vi "更新程序.vi"() -> ()   [LabVIEW 2016, in "数据传输系统-02.lvlib" / "自动更新.lvlib"]
uses:
  <vilib>/FTP/NI_FTP.lvlib
panel:
  out "同名app个数":i32
  out "对比MD5":string
  out "当前MD5":string
  out "FTP链接结束":bool
  out "updateconfiguration":T1
  out "软件版本 2":string caption="目标软件版本"
  out "软件版本":string caption="当前软件版本"
  out "下载的文件名":string
  out "目标文件夹名":string
  out "端口号":i32
  out "IP地址":string
  out "步骤":string
  out "枚举":T2(ring)
  in  "目标路径（使用对话框）":path
  out "下载保存目录":path
  out "更新进度":u8(slide) scale=0.0..100.0
  # "1.下载更新--------2.MD5校验-------2.关闭主应用-------3.替换应用--------4.打开主应用-----------5.关闭本程序"
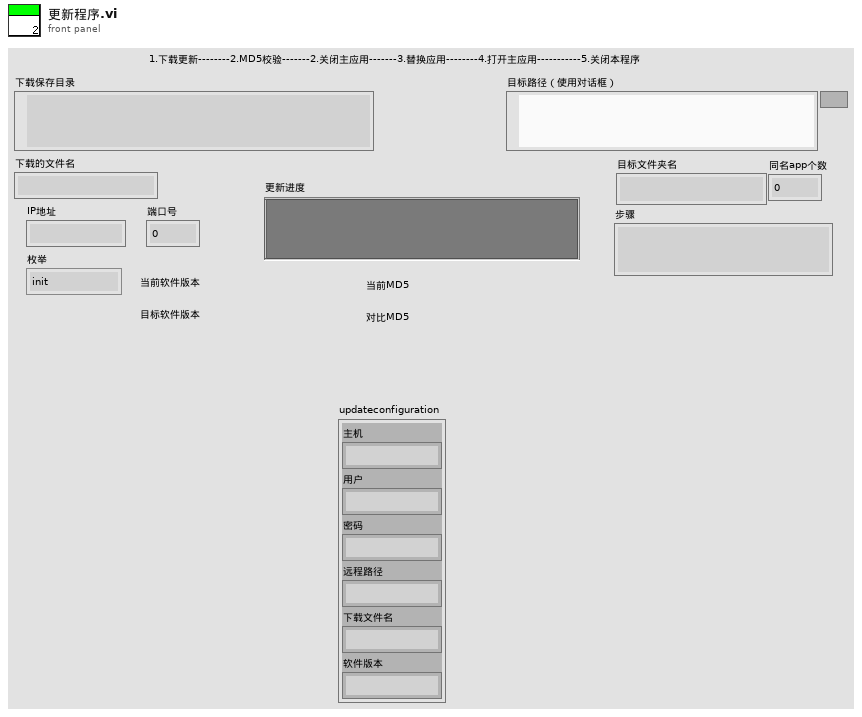
[diagram p1: front panel]
types:
  T1 = cluster{"主机":string, "用户":string, "密码":string, "远程路径":string, "下载文件名":string, "软件版本":string}
  T2 = enum16{"init", "download", "close", "replace", "open", "over"}
  T3 = typedef "NI_FTP.lvlib/FTP File Info.ctl" = cluster{"type":enum16{"unknown", "file", "dir", "link"}, "permissions":string, "owner":string, "group":string, "size":i32, "date":string, "name":string, "link name":string}
  T4 = enum16{"open", "replace", "create", "open or create", "replace or create", "replace or create with confirmation"}
  T5 = cluster{"网络灯":bool, "接收中":bool, "已接收百分比":u8, "接收成功次数":dbl, "当前步骤":enum16{"init", "receivehead", "receivecontent", "receivesuccess", "over"}, "文件名":string, "error out":errorcluster}
  T6 = cluster{"remote path":string, "local path":path, "binary":bool}
  T7 = typedef "NI_FTP.lvlib/FTP Session.ctl" = refnum<k5>
  T8 = cluster{"remote path":string, "local path":path, "binary":bool}[]
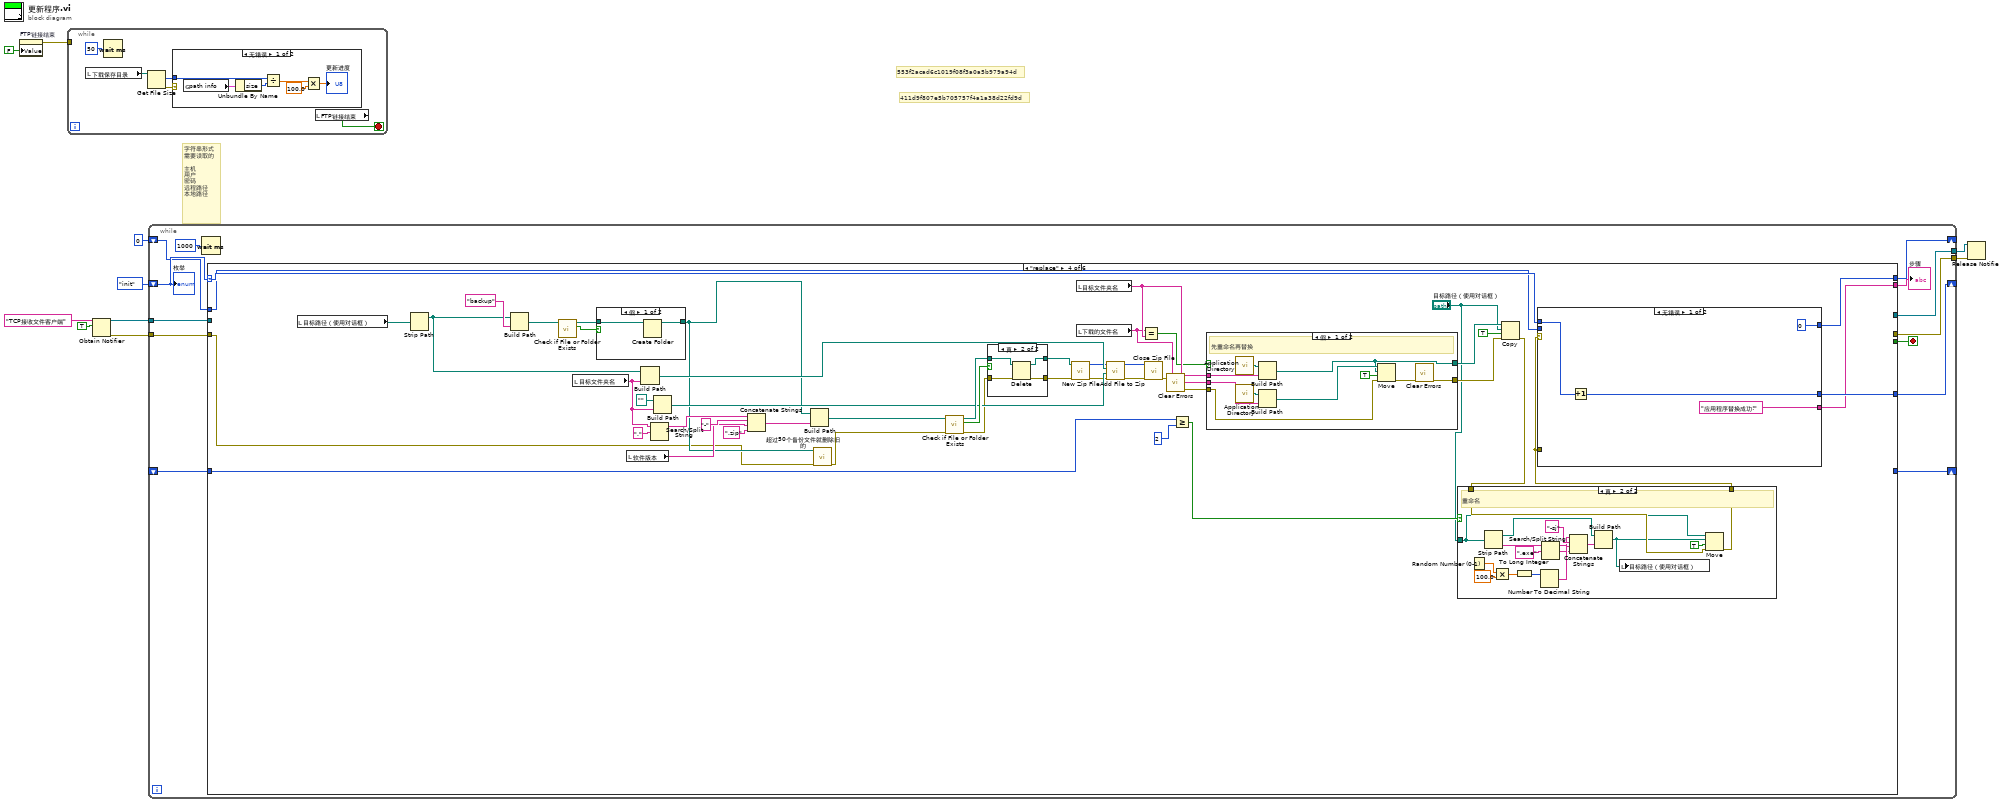
[diagram p0: block diagram]
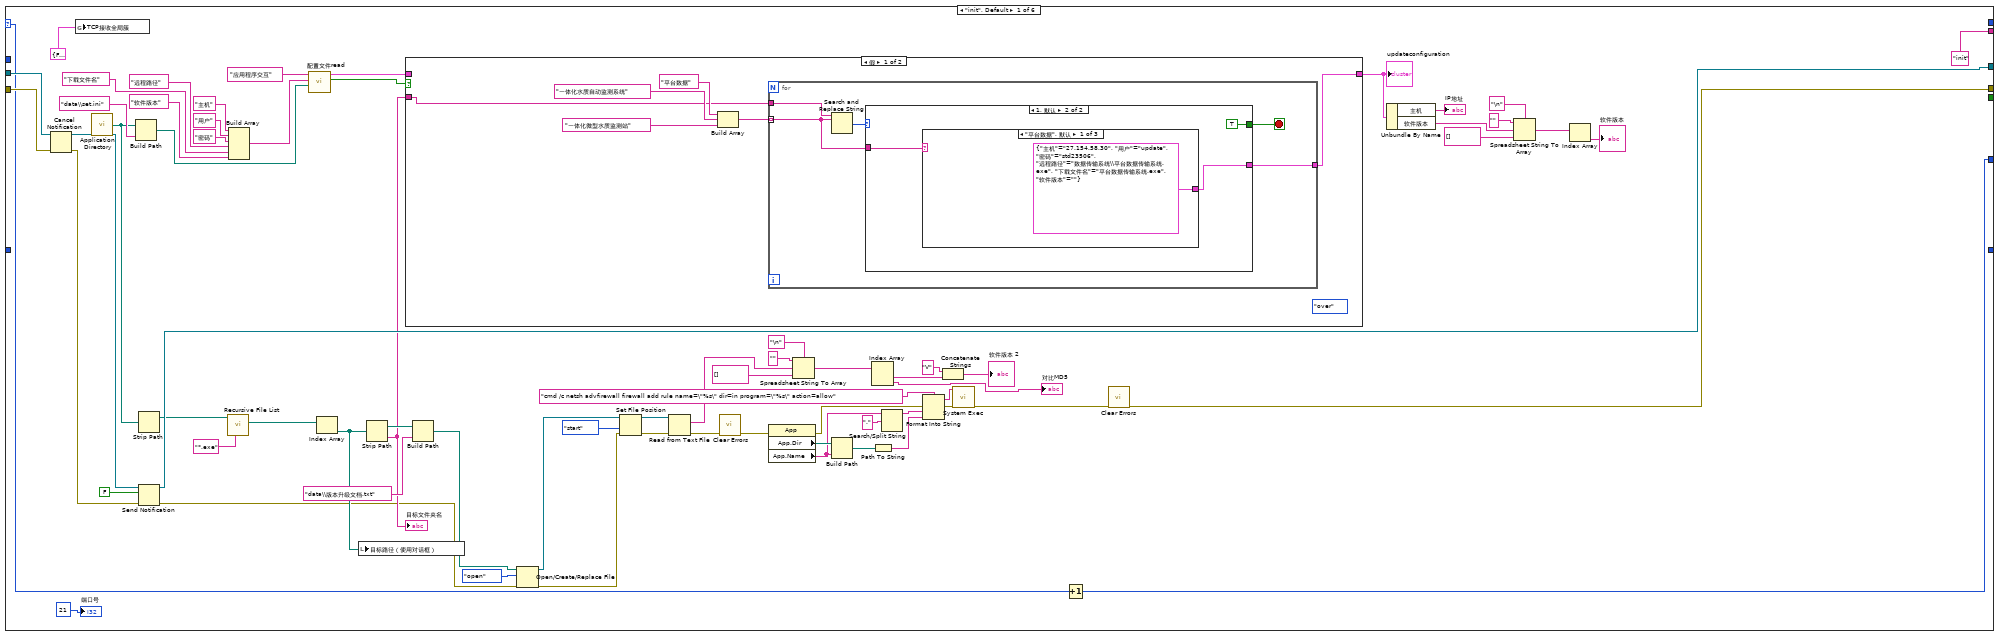
[diagram p3: hidden frame]
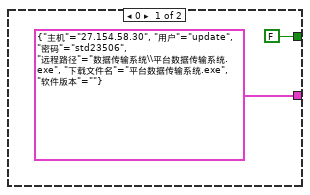
[diagram p4: hidden frame]
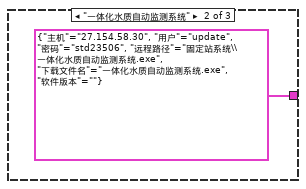
[diagram p5: hidden frame]
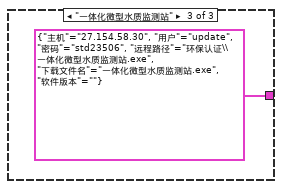
[diagram p6: hidden frame]
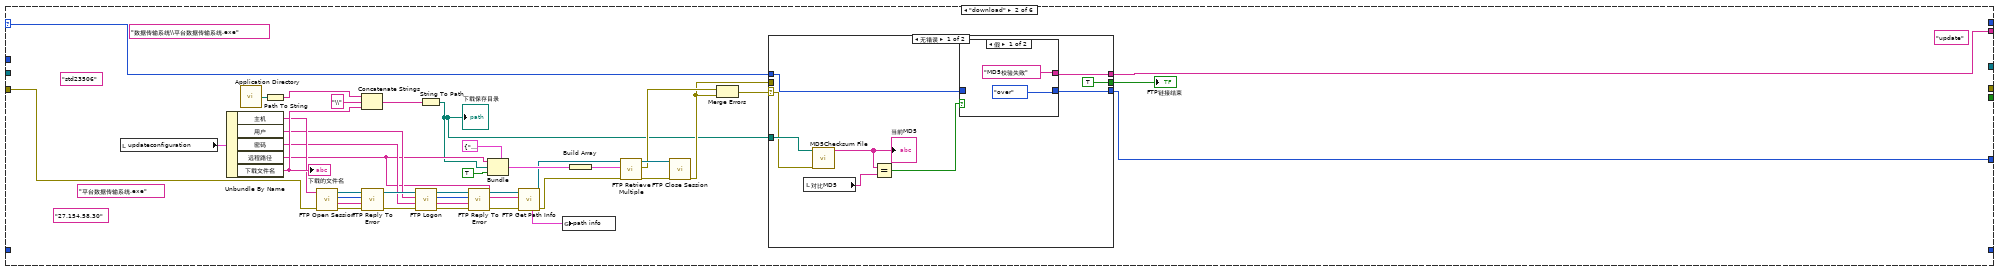
[diagram p8: hidden frame]
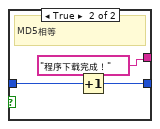
[diagram p9: hidden frame]
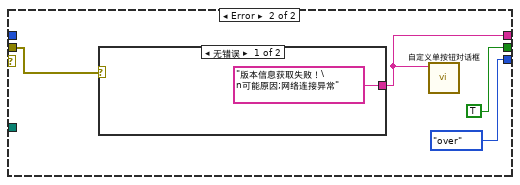
[diagram p10: hidden frame]
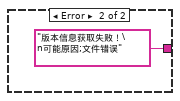
[diagram p11: hidden frame]
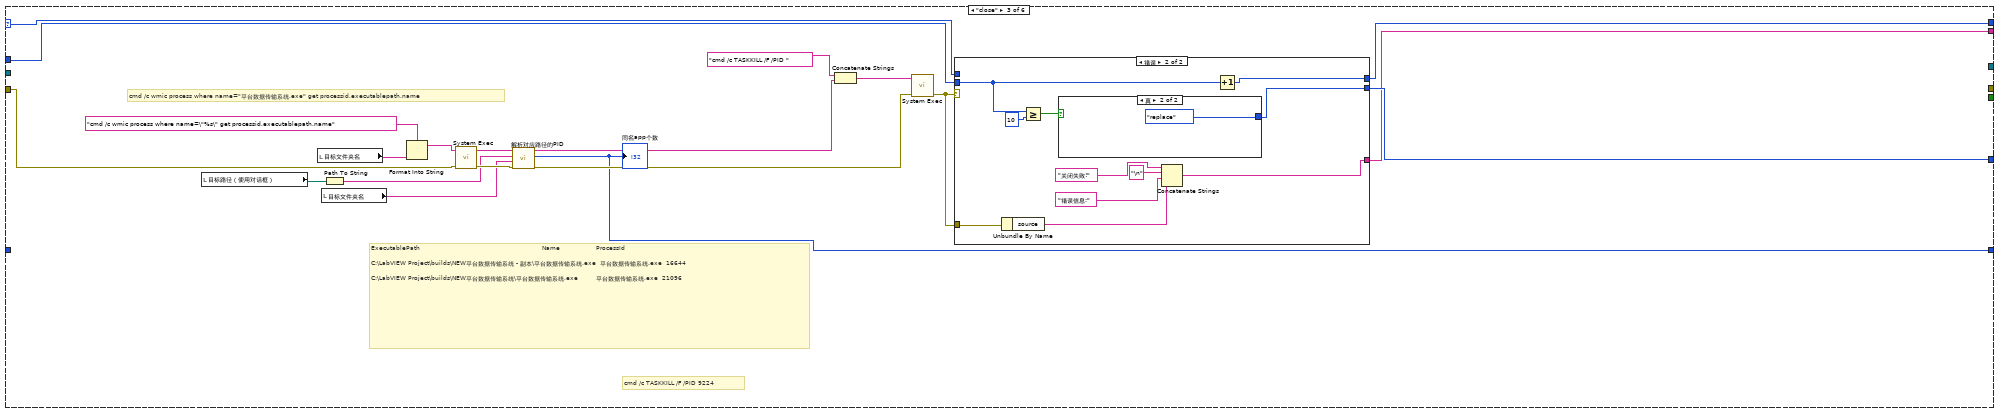
[diagram p12: hidden frame]
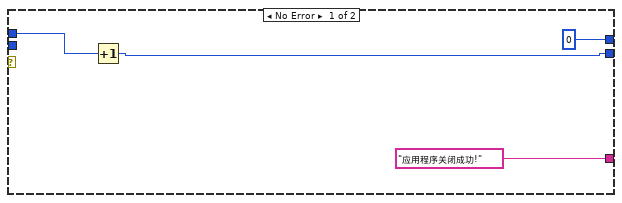
[diagram p13: hidden frame]
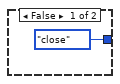
[diagram p14: hidden frame]
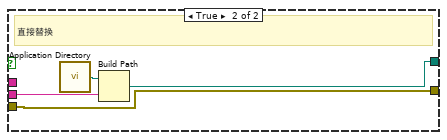
[diagram p16: hidden frame]
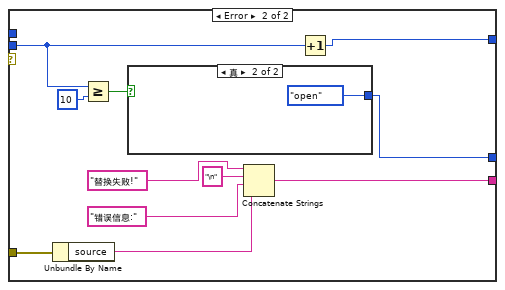
[diagram p19: hidden frame]
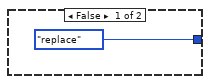
[diagram p20: hidden frame]
diagram:
  # "411d9f807e5b705757f4a1a38d22fd9d"
  # "553f2acad6c1019f08f3a0a5b979a94d"
  # "字符串形式\n需要读取的\n\n主机\n用户\n密码\n远程路径\n本地路径"
  n1 = property on="FTP链接结束" class="Bool (严格)"("Value"=FALSE ("FTP链接结束")) -> (error out=w1:errorcluster)  [unwired: 2 in, 1 out]
  n2 = while {
    tunnel: w1 -> [_]
    stop <- w15 stop-if-true
    n3 = local read "下载保存目录"() -> (w13:path)
    n4 = Wait (ms)(milliseconds to wait=u32 50 ("等待时间（毫秒）")) -> ()  [unwired: 1 out]
    n5 = Get File Size(file=w13) -> (size (in bytes)=w11:i64, 0:w12:errorcluster)  [unwired: 1 in, 1 out]
    n6 = case shown="无错误" w12 {
      tunnel: w11 -> [w17 _]
      frame No Error {
        n7 = global read "update全局.vi" "path info"() -> (w18:T3)
        n8 = Unbundle By Name(w18) -> ("size"=w21:i32)
        n9 = Divide(x=w17, y=w21) -> (x/y=w20:dbl)
        n10 = Multiply(x=w20, y=100.0) -> (x*y=→"更新进度":dbl)
      }
      frame Error {
      }
    }
    n11 = local read "FTP链接结束"() -> (w15:bool)
  }
  n12 = Obtain Notifier(name (unnamed)="TCP接收文件客户端" ("名称（未命名）"), notification data type=TRUE) -> (notifier out=w7:refnum<notifier>, error out=w6:errorcluster)  [unwired: 2 in, 1 out]
  n13 = while {
    shift-right: [w33] -> _
    shift-left: T2."init" -> [w34]
    tunnel: w7 -> [w29]
    tunnel: w6 -> [w28]
    tunnel: [w27] -> w5
    tunnel: [w26] -> w4
    shift-right: [w24] -> _
    shift-left: u8 0 -> [w25]
    shift-right: [w23] -> _
    shift-left: _ -> [w22]
    stop <- w32 stop-if-true
    n14 = Wait (ms)(milliseconds to wait=u32 1000 ("等待时间（毫秒）")) -> ()  [unwired: 1 out]
    n15 = case shown="\"replace\"" w34 {
      selector: w34 -> [w52 w162 w201 w269 _ w377]
      tunnel: [w51 w163 w200 w268 w331 w376] -> w33
      tunnel: [_ _ _ _ _ w372] -> w32
      tunnel: ["init" ("步骤") w161 w199 w267 w330 "over" ("步骤")] -> w30
      tunnel: w29 -> [w103 _ _ _ _ w374]
      tunnel: w28 -> [w102 w126 w186 w230 _ w352]
      tunnel: [w98 _ _ _ _ w373] -> w27
      tunnel: [w37 _ _ _ _ w357] -> w26
      tunnel: w25 -> [_ _ w198 w261 w328 _]
      tunnel: [_ _ w197 w260 w329 _] -> w24
      tunnel: [_ _ w185 _ _ _] -> w23
      tunnel: w22 -> [_ _ _ w226 _ _]
      frame "init", Default {
        n16 = Cancel Notification(0:w103, 3:w102) -> (8:w101:refnum<notifier>, 11:w99:errorcluster)  [unwired: 1 out]
        n17 = global write "全局变量1.vi" "TCP接收全局簇"(T5 {"网络灯"=FALSE, "接收中"=FALSE, "已接收百分比"=0, "接收成功次数"=0.0, "当前步骤"=enum."init", "文件名"="", "error out"={"status"=FALSE, "code"=0, "source"=""}} ("TCP接收全局簇")) -> ()
        n18 = call <vilib>:"Application Directory.vi"() -> ("Application Directory"=w59:path)
        n19 = Build Path(base path=w59, name or relative path="data\\set.ini" ("名称或相对路径")) -> (appended path=w62:path)
        n20 = Strip Path(path=w59) -> (stripped path=w93:path)  [unwired: 1 out]
        n21 = Send Notification(notification=FALSE ("通知"), notifier=w101, error in (no error)=w99) -> (notifier out=w98:refnum<notifier>, error out=w38:errorcluster)
        n22 = call <vilib>:"Recursive File List.vi"("pattern"="*.exe", "Folder Path"=w93) -> ("All Files in Dir"=w95:path[])  [unwired: 5 in, 4 out]
        n23 = Build Array("主机" ("section"), "用户" ("section"), "密码" ("key"), "远程路径" ("key"), "下载文件名" ("key"), "软件版本" ("key")) -> (w66:string[])
        n24 = call "配置文件read.vi"("configuration file path"=w62, "键数组"=w66, "段"="应用程序交互" ("section")) -> ("section exists?"=w68:bool, "updateconfiguration"=w69:T1)  [unwired: 6 in, 1 out]
        n25 = Index Array(array=w95) -> (element=w96:path)  [unwired: 1 in]
        n26 = local write "目标路径（使用对话框）"(w96) -> ()
        n27 = Strip Path(path=w96) -> (stripped path=w70:path, name=w53:string)
        "目标文件夹名" <- w53
        n28 = case shown="假" w68 {
          tunnel: w69 -> [_ w124]
          tunnel: [w105 w124] -> w61
          tunnel: w53 -> [w106 _]
          frame False {
            (unwired) T2."over"
            n29 = Build Array("平台数据" ("搜索字符串"), "一体化水质自动监测系统" ("搜索字符串"), "一体化微型水质监测站" ("搜索字符串")) -> (w107:string[])
            n30 = for {
              tunnel: w107 -> [w112] mode=indexing
              tunnel: w106 -> [w113]
              tunnel: [w111] -> w105
              stop <- w114 stop-if-true
              n31 = Search and Replace String(input string=w113, search string=w112) -> (number of replacements=w115:i32)  [unwired: 6 in, 3 out]
              n32 = case shown="1, 默认" w115 {
                tunnel: [FALSE TRUE] -> w114
                tunnel: w112 -> [_ w119]
                tunnel: [T1 {"主机"="27.154.58.30", "用户"="update", "密码"="std23506", "远程路径"="数据传输系统\\平台数据传输系统.exe", "下载文件名"="平台数据传输系统.exe", "软件版本"=""} ("updateconfiguration") w118] -> w111
                frame 0 {
                }
                frame 1, Default {
                  n33 = case shown="\"平台数据\", 默认" w119 {
                    tunnel: [T1 {"主机"="27.154.58.30", "用户"="update", "密码"="std23506", "远程路径"="数据传输系统\\平台数据传输系统.exe", "下载文件名"="平台数据传输系统.exe", "软件版本"=""} ("updateconfiguration") T1 {"主机"="27.154.58.30", "用户"="update", "密码"="std23506", "远程路径"="固定站系统\\一体化水质自动监测系统.exe", "下载文件名"="一体化水质自动监测系统.exe", "软件版本"=""} ("updateconfiguration") T1 {"主机"="27.154.58.30", "用户"="update", "密码"="std23506", "远程路径"="环保认证\\一体化微型水质监测站.exe", "下载文件名"="一体化微型水质监测站.exe", "软件版本"=""} ("updateconfiguration")] -> w118
                    frame "平台数据", Default {
                    }
                    frame "一体化水质自动监测系统" {
                    }
                    frame "一体化微型水质监测站" {
                    }
                  }
                }
              }
            }
          }
          frame True {
          }
        }
        "updateconfiguration" <- w61
        n34 = Build Path(base path=w70, name or relative path="data\\版本升级文档.txt" ("名称或相对路径")) -> (appended path=w78:path)
        n35 = Open/Create/Replace File(file path (use dialog)=w78, error in=w38, operation (0:open)=T4."open" ("操作(0:open)")) -> (refnum out=w73:refnum<file>, error out=w74:errorcluster)  [unwired: 3 in, 1 out]
        n36 = Set File Position(refnum=w73, from (0:start)=enum16{"start", "end", "current"}."start" ("自（0:起始）"), error in=w74) -> (refnum out=w77:refnum<file>, error out=w75:errorcluster)  [unwired: 1 in]
        n37 = Read from Text File(file (use dialog)=w77, error in=w75) -> (text=w85:string, error out=w42:errorcluster)  [unwired: 2 in, 2 out]
        n38 = call <vilib>:"Clear Errors.vi"("error in (no error)"=w42) -> ("error out"=w36:errorcluster)  [unwired: 5 in, 1 out]
        n39 = property class="App"(error in=w36) -> (error out=w41:errorcluster, "App.Dir"=w50:path, "App.Name"=w45:string)  [unwired: 1 in, 1 out]
        n40 = Spreadsheet String To Array(delimiter (Tab)="\n" ("分隔符(Tab)"), format string="" ("格式字符串"), spreadsheet string=w85, array type (2D Dbl)=string[] []) -> (array=w82:string[])
        n41 = Build Path(base path=w50, name or relative path=w45) -> (appended path=w49:path)
        n42 = Index Array(array=w82) -> (element #1=w83:string, element #2=→"对比MD5":string)  [unwired: 2 in]
        n43 = Path To String(path=w49) -> (string=w47:string)
        n44 = Search/Split String(string=w45, search string/char (-)="." ("搜索字符串/字符(-)")) -> (substring before match=w44:string)  [unwired: 1 in, 2 out]
        n45 = Format Into String(format string="cmd /c netsh advfirewall firewall add rule name=\"%s\" dir=in program=\"%s\" action=allow" ("command line"), error in=w41, w44, w47) -> (resulting string=w43:string, error out=w40:errorcluster)  [unwired: 1 in]
        n46 = Concatenate Strings("V" ("字符串"), w83) -> (→"软件版本 2":string)
        n47 = call <vilib>:"System Exec.vi"("error in (no error)"=w40, "command line"=w43) -> ("error out"=w39:errorcluster)  [unwired: 6 in, 3 out]
        n48 = Increment(x=w52) -> (x+1=w51:T2)
        n49 = call <vilib>:"Clear Errors.vi"("error in (no error)"=w39) -> ("error out"=w37:errorcluster)  [unwired: 5 in, 1 out]
        n50 = Unbundle By Name(w61) -> ("主机"=→"IP地址":string, "软件版本"=w54:string)
        n51 = Spreadsheet String To Array(delimiter (Tab)="\n" ("分隔符(Tab)"), format string="" ("格式字符串"), spreadsheet string=w54, array type (2D Dbl)=string[] []) -> (array=w88:string[])
        n52 = Index Array(array=w88) -> (element=→"软件版本":string)  [unwired: 1 in]
        "端口号" <- 21 ("端口号")
      }
      frame "download" {
        (unwired) "平台数据传输系统.exe" ("字符串")
        (unwired) "std23506" ("password")
        (unwired) "update" ("user")
        (unwired) "数据传输系统\\平台数据传输系统.exe" ("remote path")
        (unwired) "27.154.58.30" ("host")
        n53 = local read "updateconfiguration"() -> (w157:T1)
        n54 = Unbundle By Name(w157) -> ("主机"=w142:string, "用户"=w141:string, "密码"=w140:string, "远程路径"=w137:string, "下载文件名"=w155:string)
        "下载的文件名" <- w155
        n55 = call <vilib>:"Application Directory.vi"() -> ("Application Directory"=w160:path)
        n56 = Path To String(path=w160) -> (string=w159:string)
        n57 = call <vilib>:"FTP Open Session.vi"("error in (no error)"=w126, "address"=w142) -> ("error out"=w144:errorcluster, "reply string"=w146:string, "reply code"=w145:i32, "ftp session"=w143:T7)  [unwired: 2 in, 4 out]
        n58 = Concatenate Strings(w159, "\\" ("字符串"), w155) -> (w158:string)
        n59 = call <vilib>:"FTP Reply To Error.vi"("error in (no error)"=w144, "reply string in"=w146, "reply code in"=w145, "ftp session"=w143) -> ("error out"=w147:errorcluster, "ftp session out"=w148:T7)  [unwired: 2 out]
        n60 = call <vilib>:"FTP Logon.vi"("error in (no error)"=w147, "password"=w140, "user"=w141, "ftp session"=w148) -> ("error out"=w149:errorcluster, "reply string"=w151:string, "reply code"=w152:i32, "ftp session out"=w150:T7)  [unwired: 4 out]
        n61 = String To Path(string=w158) -> (path=w125:path)
        "下载保存目录" <- w125
        n62 = call <vilib>:"FTP Reply To Error.vi"("error in (no error)"=w149, "reply string in"=w151, "reply code in"=w152, "ftp session"=w150) -> ("error out"=w154:errorcluster, "ftp session out"=w153:T7)  [unwired: 2 out]
        n63 = Bundle(cluster=T6 {"remote path"="", "local path"=path "", "binary"=FALSE} ("transfer spec"), "remote path"=w137, "local path"=w125, "binary"=TRUE) -> (w139:T6)
        n64 = call <vilib>:"FTP Get Path Info.vi"("error in (no error)"=w154, "remote path"=w137, "ftp session"=w153) -> ("error out"=w133:errorcluster, "ftp session out"=w135:T7, "path info"=w134:T3)  [unwired: 4 in, 2 out]
        n65 = global write "update全局.vi" "path info"(w134) -> ()
        n66 = Build Array(w139) -> (w132:T8)
        n67 = call <vilib>:"FTP Retrieve Multiple.vi"("error in (no error)"=w133, "file specifications"=w132, "ftp session"=w135) -> ("error out"=w130:errorcluster, "file errors"=w129:errorcluster[], "ftp session out"=w131:T7)  [unwired: 2 in, 4 out]
        n68 = call <vilib>:"FTP Close Session.vi"("error in (no error)"=w130, "ftp session"=w131) -> ("error out"=w128:errorcluster)  [unwired: 9 out]
        n69 = Merge Errors(w129, w128) -> (w164:errorcluster)
        n70 = case shown="无错误" w164 {
          selector: w164 -> [w168 _]
          tunnel: w128 -> [_ w182]
          tunnel: [w173 T2."over"] -> w163
          tunnel: w162 -> [w172 _]
          tunnel: [w171 w180] -> w161
          tunnel: [TRUE ("FTP链接结束") TRUE ("FTP链接结束")] -> w127
          tunnel: w125 -> [w169 _]
          frame No Error {
            n71 = local read "对比MD5"() -> (w166:string)
            n72 = call <vilib>:"MD5Checksum File.vi"("error in (no error)"=w168, "Path"=w169) -> ("MD5 message-digest"=w167:string)  [unwired: 8 in, 1 out]
            "当前MD5" <- w167
            n73 = Equal?(x=w167, y=w166) -> (x = y?=w165:bool)
            n74 = case shown="假" w165 {
              tunnel: [T2."over" w178] -> w173
              tunnel: w172 -> [_ w177]
              tunnel: ["MD5校验失败" "程序下载完成！"] -> w171
              frame False {
              }
              frame True {
                # "MD5相等"
                n75 = Increment(x=w177) -> (x+1=w178:T2)
              }
            }
          }
          frame Error {
            n76 = case shown="无错误" w182 {
              tunnel: ["版本信息获取失败！\n可能原因;网络连接异常" "版本信息获取失败！\n可能原因;文件错误"] -> w180
              frame No Error {
              }
              frame Error {
              }
            }
            n77 = call "自定义单按钮对话框.vi"("消息"=w180) -> ()  [unwired: 11 in]
          }
        }
        "FTP链接结束" <- w127
      }
      frame "close" {
        # "cmd /c TASKKILL /F /PID 9224"
        # "ExecutablePath                                                             Name                  ProcessId  \n\nC:\\LabVIEW Project\\builds\\NEW平台数据传输系统 - 副本\\平台数据传输系统.exe  平台数据传输系统.exe  16644      \n\nC:\\LabVIEW Project\\builds\\NEW平台数据传输系统\\平台数据传输系统.exe         平台数据传输系统.exe  21096"
        # "cmd /c wmic process where name=\"平台数据传输系统.exe\" get processid,executablepath,name"
        n78 = local read "目标路径（使用对话框）"() -> (w191:path)
        n79 = local read "目标文件夹名"() -> (w195:string)
        n80 = local read "目标文件夹名"() -> (w189:string)
        n81 = Path To String(path=w191) -> (string=w190:string)
        n82 = Format Into String(format string="cmd /c wmic process where name=\"%s\" get processid,executablepath,name" ("command line"), w195) -> (resulting string=w194:string)  [unwired: 2 in, 1 out]
        n83 = call <vilib>:"System Exec.vi"("error in (no error)"=w186, "command line"=w194) -> ("error out"=w192:errorcluster, "standard output"=w193:string)  [unwired: 6 in, 2 out]
        n84 = call "解析对应路径的PID.vi"("error in (no error)"=w192, "appname"=w189, "Path"=w190, "输入"=w193) -> ("error out"=w187:errorcluster, "同名app个数"=w185:i32, "PID"=w188:string)  [unwired: 5 in]
        "同名app个数" <- w185
        n85 = Concatenate Strings("cmd /c TASKKILL /F /PID " ("command line"), w188) -> (w202:string)
        n86 = call <vilib>:"System Exec.vi"("error in (no error)"=w187, "command line"=w202) -> ("error out"=w204:errorcluster)  [unwired: 6 in, 3 out]
        n87 = case shown="错误" w204 {
          tunnel: [w206 w213] -> w200
          tunnel: w204 -> [_ w219]
          tunnel: ["应用程序关闭成功!" ("步骤") w214] -> w199
          tunnel: w201 -> [w207 _]
          tunnel: w198 -> [_ w209]
          tunnel: [u8 0 w211] -> w197
          frame No Error {
            n88 = Increment(x=w207) -> (x+1=w206:T2)
          }
          frame Error {
            n89 = Unbundle By Name(w219) -> ("source"=w218:string)
            n90 = Greater Or Equal?(x=w209, y=u8 10) -> (x >= y?=w210:bool)
            n91 = case shown="真" w210 {
              tunnel: [T2."close" T2."replace"] -> w213
              frame False {
              }
              frame True {
              }
            }
            n92 = Concatenate Strings("关闭失败!" ("消息"), "\n" ("字符串"), "错误信息:" ("字符串"), w218) -> (w214:string)
            n93 = Increment(x=w209) -> (x+1=w211:u8)
          }
        }
      }
      frame "replace" {
        n94 = local read "目标路径（使用对话框）"() -> (w238:path)
        n95 = Strip Path(path=w238) -> (stripped path=w237:path)  [unwired: 1 out]
        n96 = Build Path(base path=w237, name or relative path="backup" ("名称或相对路径")) -> (appended path=w253:path)
        n97 = call <vilib>:"Check if File or Folder Exists.vi"("path"=w253) -> ("file or folder exists?"=w254:bool, "dup path"=w255:path)  [unwired: 8 in, 1 out]
        n98 = local read "目标文件夹名"() -> (w236:string)
        n99 = case shown="假" w254 {
          tunnel: w255 -> [w309 w310]
          tunnel: [w308 w310] -> w231
          frame False {
            n100 = Create Folder(path (use dialog)=w309) -> (created path=w308:path)  [unwired: 2 in, 2 out]
          }
          frame True {
          }
        }
        n101 = local read "软件版本"() -> (w239:string)
        n102 = Build Path(base path=w237, name or relative path=w236) -> (appended path=w250:path)
        n103 = Search/Split String(string=w236, search string/char (-)="." ("搜索字符串/字符(-)")) -> (substring before match=w244:string)  [unwired: 1 in, 2 out]
        n104 = Build Path(base path=path "" ("Relative Path from 1 to 2"), name or relative path=w236) -> (appended path=w252:path)
        n105 = Concatenate Strings(w244, "-" ("字符串"), w239, ".zip" ("字符串")) -> (w245:string)
        n106 = Build Path(base path=w231, name or relative path=w245) -> (appended path=w232:path)
        n107 = call "超过50个备份文件就删除旧的.vi"("error in (no error)"=w230, "Folder Path"=w231) -> ("error out"=w229:errorcluster)  [unwired: 9 in]
        n108 = call <vilib>:"Check if File or Folder Exists.vi"("error in (no error)"=w229, "path"=w232) -> ("error out"=w234:errorcluster, "file or folder exists?"=w257:bool, "dup path"=w256:path)  [unwired: 7 in]
        n109 = case shown="真" w257 {
          tunnel: w256 -> [w303 w307]
          tunnel: [w303 w306] -> w258
          tunnel: w234 -> [w302 w305]
          tunnel: [w302 w304] -> w233
          frame False {
          }
          frame True {
            n110 = Delete(path (use dialog)=w307, error in=w305) -> (deleted path=w306:path, error out=w304:errorcluster)  [unwired: 3 in, 1 out]
          }
        }
        n111 = call <vilib>:"New Zip File.vi"("error in (no error)"=w233, "target"=w258) -> ("error out"=w246:errorcluster, "zip file out"=w247:i64)  [unwired: 1 in, 3 out]
        n112 = local read "目标文件夹名"() -> (w264:string)
        n113 = local read "下载的文件名"() -> (w263:string)
        n114 = call <vilib>:"Add File to Zip.vi"("error in (no error)"=w246, "destination path in zip"=w252, "source file path"=w250, "zip file in"=w247) -> ("error out"=w249:errorcluster, "zip file out"=w248:i64)  [unwired: 6 in]
        n115 = Equal?(x=w263, y=w264) -> (x = y?=w262:bool)
        n116 = call <vilib>:"Close Zip File.vi"("error in (no error)"=w249, "zip file in"=w248) -> ("error out"=w235:errorcluster)  [unwired: 5 in]
        n117 = call <vilib>:"Clear Errors.vi"("error in (no error)"=w235) -> ("error out"=w228:errorcluster)  [unwired: 5 in, 1 out]
        n118 = Greater Or Equal?(x=w226, y=2) -> (x >= y?=w223:bool)
        n119 = case shown="假" w262 {
          tunnel: w263 -> [w294 w300]
          tunnel: w264 -> [w293 _]
          tunnel: [w292 w299] -> w266
          tunnel: [w289 w298] -> w259
          tunnel: w228 -> [w288 w298]
          frame False {
            # "先重命名再替换"
            n120 = call <vilib>:"Application Directory.vi"() -> ("Application Directory"=w296:path)
            n121 = call <vilib>:"Application Directory.vi"() -> ("Application Directory"=w295:path)
            n122 = Build Path(base path=w296, name or relative path=w293) -> (appended path=w292:path)
            n123 = Build Path(base path=w295, name or relative path=w294) -> (appended path=w297:path)
            n124 = Move(source path=w297, error in=w288, 9:TRUE ("覆盖(F)"), 10:w292) -> (error out=w290:errorcluster)  [unwired: 1 in, 2 out]
            n125 = call <vilib>:"Clear Errors.vi"("error in (no error)"=w290) -> ("error out"=w289:errorcluster)  [unwired: 5 in, 1 out]
          }
          frame True {
            # "直接替换"
            n126 = call <vilib>:"Application Directory.vi"() -> ("Application Directory"=w301:path)
            n127 = Build Path(base path=w301, name or relative path=w300) -> (appended path=w299:path)
          }
        }
        n128 = Copy(8:w259, 9:TRUE ("覆盖(F)"), 10:"目标路径（使用对话框）", 11:w266) -> (0:w225:errorcluster)  [unwired: 1 in, 2 out]
        n129 = case shown="真" w223 {
          tunnel: w225 -> [w270 w286]
          tunnel: [w270 w285] -> w224
          tunnel: "目标路径（使用对话框）" -> [_ w284]
          frame False {
            # "不重命名"
          }
          frame True {
            # "重命名"
            n130 = Random Number (0-1)() -> (number: 0 to 1=w278:dbl)
            n131 = Strip Path(path=w284) -> (stripped path=w283:path, name=w271:string)
            n132 = Multiply(x=w278, y=100.0) -> (x*y=w280:dbl)
            n133 = To Long Integer(number=w280) -> (32bit integer=w281:i32)
            n134 = Number To Decimal String(number=w281) -> (decimal integer string=w277:string)  [unwired: 1 in]
            n135 = Search/Split String(string=w271, search string/char (-)=".exe" ("搜索字符串/字符(-)")) -> (substring before match=w275:string, match + rest of string=w274:string)  [unwired: 1 in, 1 out]
            n136 = Concatenate Strings(w275, "-sj" ("字符串"), w277, w274) -> (w273:string)
            n137 = Build Path(base path=w283, name or relative path=w273) -> (appended path=w272:path)
            n138 = local write "目标路径（使用对话框）"(w272) -> ()
            n139 = Move(source path=w284, error in=w286, 9:TRUE ("覆盖(F)"), 10:w272) -> (error out=w285:errorcluster)  [unwired: 1 in, 2 out]
          }
        }
        n140 = case shown="无错误" w224 {
          tunnel: [w312 w319] -> w268
          tunnel: w224 -> [_ w325]
          tunnel: ["应用程序替换成功!" ("步骤") w320] -> w267
          tunnel: w269 -> [w313 _]
          tunnel: w261 -> [_ w317]
          tunnel: [u8 0 w315] -> w260
          frame No Error {
            n141 = Increment(x=w313) -> (x+1=w312:T2)
          }
          frame Error {
            n142 = Unbundle By Name(w325) -> ("source"=w324:string)
            n143 = Greater Or Equal?(x=w317, y=u8 10) -> (x >= y?=w316:bool)
            n144 = case shown="真" w316 {
              tunnel: [T2."replace" T2."open"] -> w319
              frame False {
              }
              frame True {
              }
            }
            n145 = Concatenate Strings("替换失败!" ("消息"), "\n" ("字符串"), "错误信息:" ("字符串"), w324) -> (w320:string)
            n146 = Increment(x=w317) -> (x+1=w315:u8)
          }
        }
      }
      frame "open" {
        n147 = local read "目标路径（使用对话框）"() -> (w332:path)
        n148 = Path To String(path=w332) -> (string=w335:string)
        n149 = call <vilib>:"System Exec.vi"("wait until completion? (T)"=FALSE, "command line"=w335) -> ("error out"=w333:errorcluster)  [unwired: 6 in, 3 out]
        n150 = case shown="错误" w333 {
          tunnel: [T2."over" w343] -> w331
          tunnel: w333 -> [_ w349]
          tunnel: ["应用程序打开成功!" ("步骤") w344] -> w330
          tunnel: w328 -> [_ w341]
          tunnel: [u8 0 w339] -> w329
          frame No Error {
          }
          frame Error {
            n151 = Unbundle By Name(w349) -> ("source"=w348:string)
            n152 = Greater Or Equal?(x=w341, y=u8 10) -> (x >= y?=w340:bool)
            n153 = case shown="假" w340 {
              tunnel: [T2."open" T2."over"] -> w343
              frame False {
              }
              frame True {
              }
            }
            n154 = Increment(x=w341) -> (x+1=w339:u8)
            n155 = Concatenate Strings("打开失败!" ("消息"), "\n" ("字符串"), "错误信息:" ("字符串"), w348) -> (w344:string)
          }
        }
      }
      frame "over" {
        w372 = TRUE
        n156 = local read "软件版本 2"() -> (w354:string)
        n157 = local read "软件版本"() -> (w356:string)
        n158 = Concatenate Strings("更新完成！\n更新前版本号:" ("字符串"), w356, "\r", "更新后版本号:", w354, "\r") -> (w370:string)
        n159 = Build Array(w370) -> (w369:string[])
        n160 = call <vilib>:"Application Directory.vi"() -> ("Application Directory"=w367:path)
        n161 = call "更新log记录.vi"("路径"=w367, "错误输入（无错误）"=w352, "logname"="版本更新log", "数组"=w369) -> ("错误输出"=w365:errorcluster)  [unwired: 7 in]
        n162 = call <vilib>:"Clear Errors.vi"("error in (no error)"=w365) -> ("error out"=w364:errorcluster)  [unwired: 5 in, 1 out]
        n163 = Increment(x=w377) -> (x+1=w376:T2)
        n164 = Send Notification(notification=w372, notifier=w374, error in (no error)=w364) -> (notifier out=w373:refnum<notifier>, error out=w360:errorcluster)
        n165 = Current VI's Path() -> (path=w362:path)
        n166 = Open VI Reference(vi path=w362, error in (no error)=w360) -> (vi reference=w361:refnum<vi>, error out=w363:errorcluster)  [unwired: 4 in]
        n167 = invoke class="VI" method="FP.Close"(reference=w361, error in=w363) -> (reference out=w358:refnum<vi>, error out=w359:errorcluster)  [unwired: 1 in, 1 out]
        n168 = Close Reference(reference=w358, error in (no error)=w359) -> (error out=w357:errorcluster)
      }
    }
    "步骤" <- w30
    "枚举" <- w34
  }
  n169 = Release Notifier(notifier=w5, error in (no error)=w4) -> ()  [unwired: 1 in, 3 out]
